vi "bmd101Parser_v1.3.vi"() -> ()   [LabVIEW 2016]
doc: "This example performs writes and reads on a serial port, as directed by the user. You can press the Write and Read buttons, and change the Read Count, while the example is running.\n\nThe parameters set for the serial port must match the parameters of the connected instrument or device. In this example, the Read Count parameter specifies the number of bytes that the serial port reads. If there were more bytes at the port than the specified number, those bytes would not be read. If there were less bytes at the port than the specified number, you would receive a timeout error.\n\nThis example expands upon the flow control options for XON and XOFF, allowing the user to choose those control characters. Also, the user can enable or disable a termination character. Some devices require a termination character in order to identify the end of command strings. Some devices send a termination character to signify the end of data to be read. This example shows how you can end the Read operation once a termination character is detected in the buffer and/or append a termination character at the end of the Write data."
uses:
  C:/Program Files/National Instruments/LabVIEW 2016/examples/Instrument IO/Serial/support/Serial - Settings.ctl
  <vilib>/Instr/_visa.llb/VISA Configure Serial Port (Instr).vi
panel:
  out "Serial Settings:Number of Bytes at Serial Port":u32
  out "size(s)":i32
  out "return count":u32
  in  "Read Count":u32=960
  out "Poor Sensor Quality: \nSensor off":bool
  out "Poor Sensor Quality: \nSensor on":bool
  out "Heart Rate":u16[](array[numeric])
  out "Heart Rate":u8[](graph)
  out "ECG":i16(graph)
  out "Stop Loop":bool
  out "Loop index":i32
  in  "Stop":bool
  in  "Serial Settings":T1={"baud rate"=57600, "data bits"=8, "parity"=enum."None", "stop bits"=10, "flow control"=0} {"flow control" items=["None"=0, "XON/XOFF"=1, "RTS/CTS"=2, "DTR/DSR"=4]; "stop bits" items=["1.0"=10, "1.5"=15, "2.0"=20]; "data bits" min=5 max=8 step=1; "baud rate" items=["75"=75, "110"=110, "134"=134, "150"=150, "300"=300, "600"=600, "1200"=1200, "1800"=1800, "2400"=2400, "4800"=4800, "7200"=7200, "9600"=9600, "14400"=14400, "19200"=19200, "28800"=28800, "38400"=38400, "56000"=56000, "57600"=57600, "115200"=115200, "128000"=128000, "230400"=230400]}
  in  "VISA resource name":refnum<visa-resource-name>="bmd101"
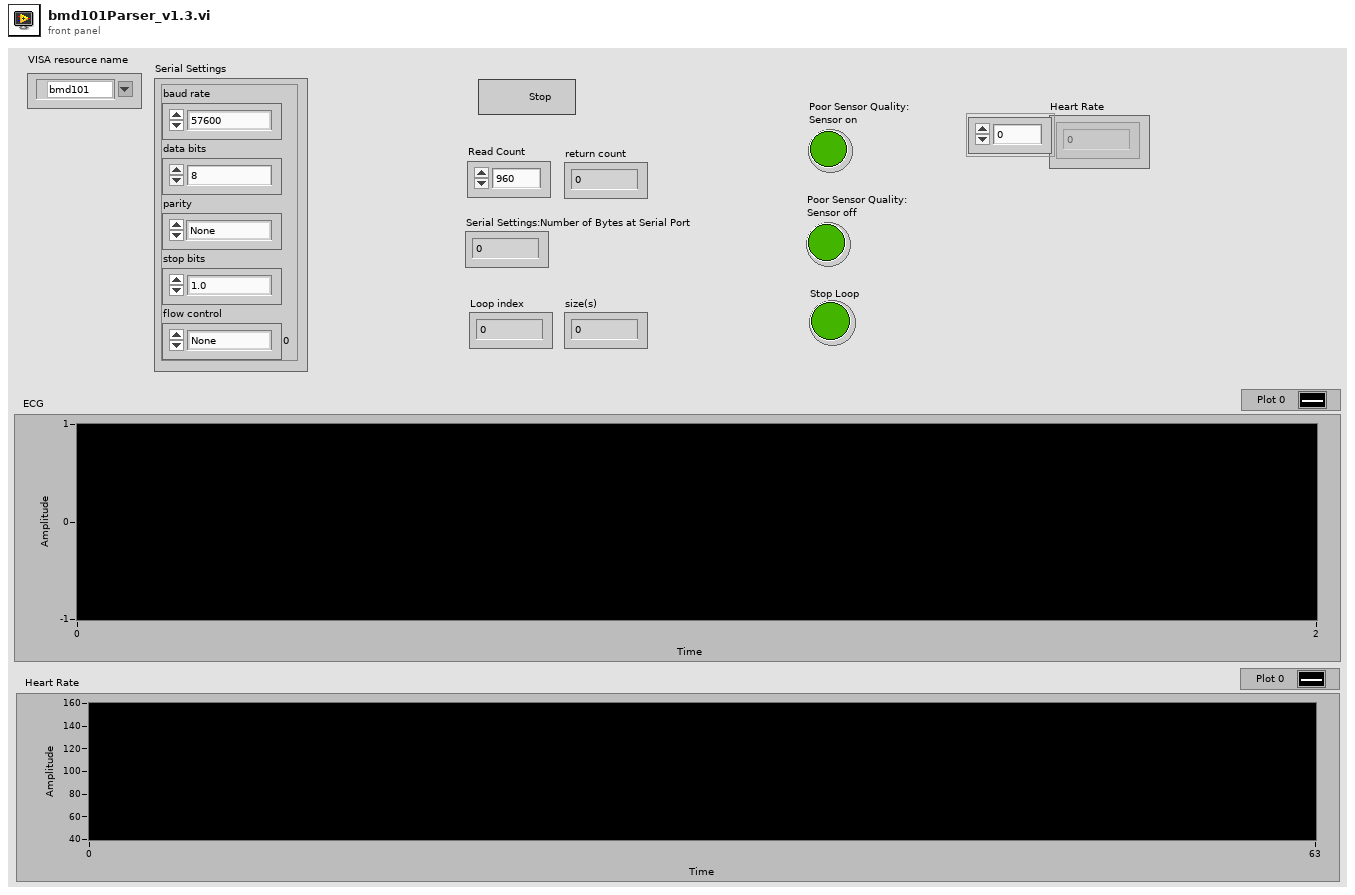
[diagram p1: front panel]
types:
  T1 = typedef "Serial - Settings.ctl" = cluster{"baud rate":u32, "data bits":u16, "parity":enum16{"None", "Odd", "Even", "Mark", "Space"}, "stop bits":u16, "flow control":u16}
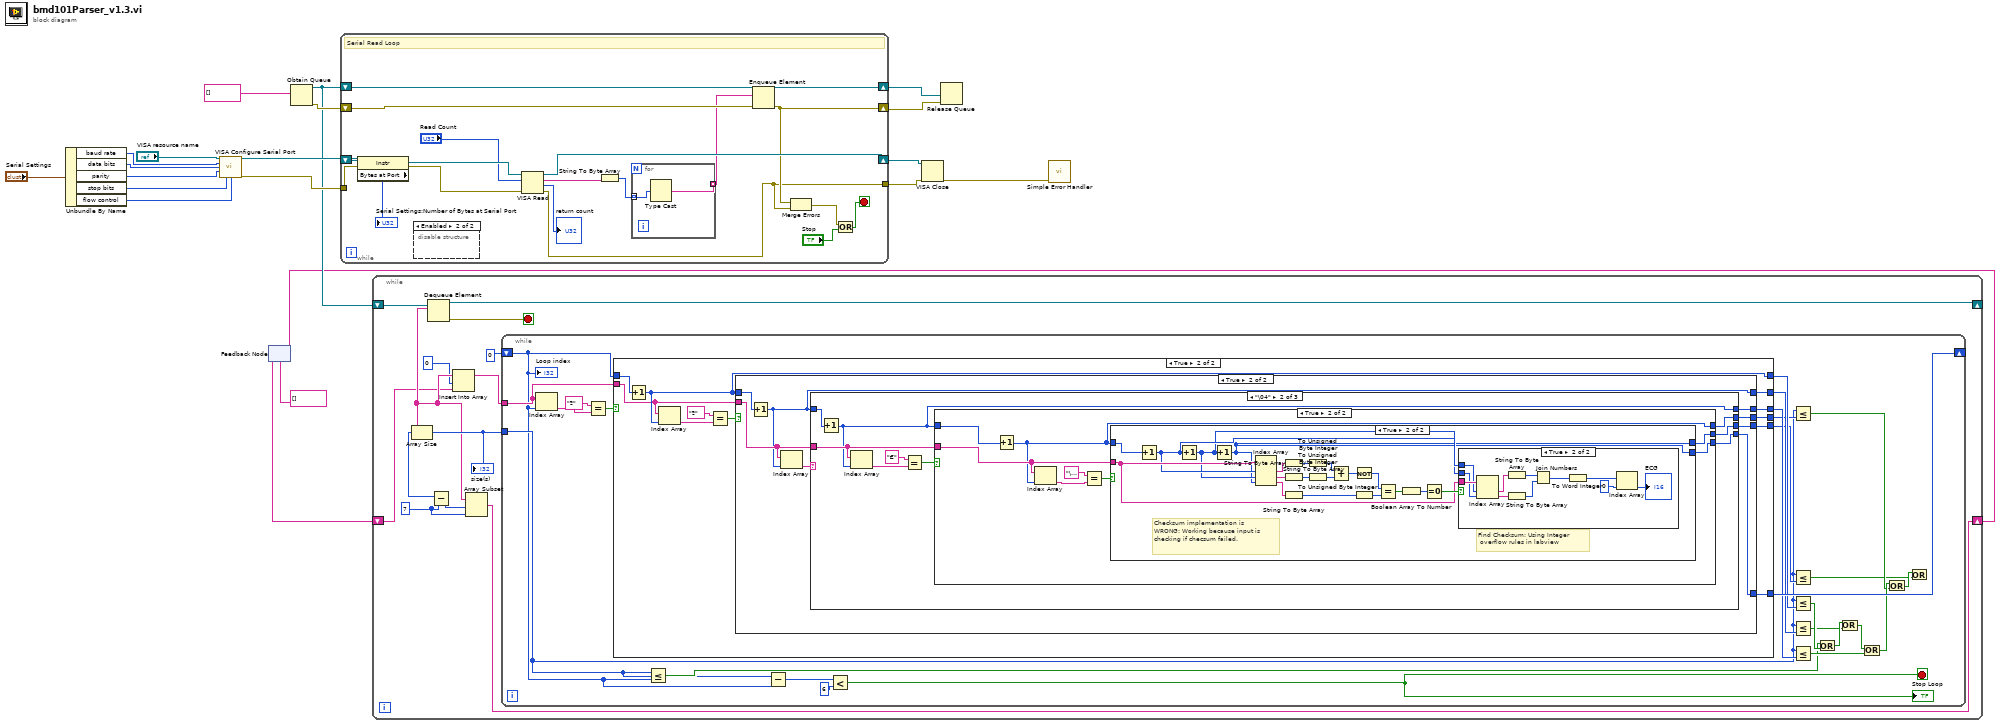
[diagram p0: block diagram]
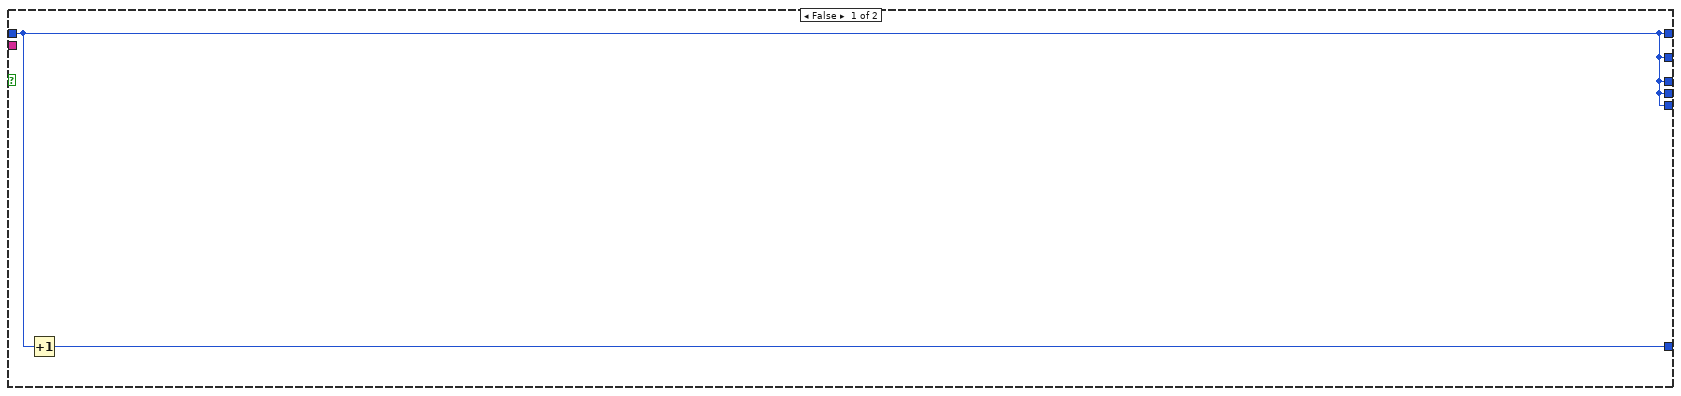
[diagram p2: hidden frame]
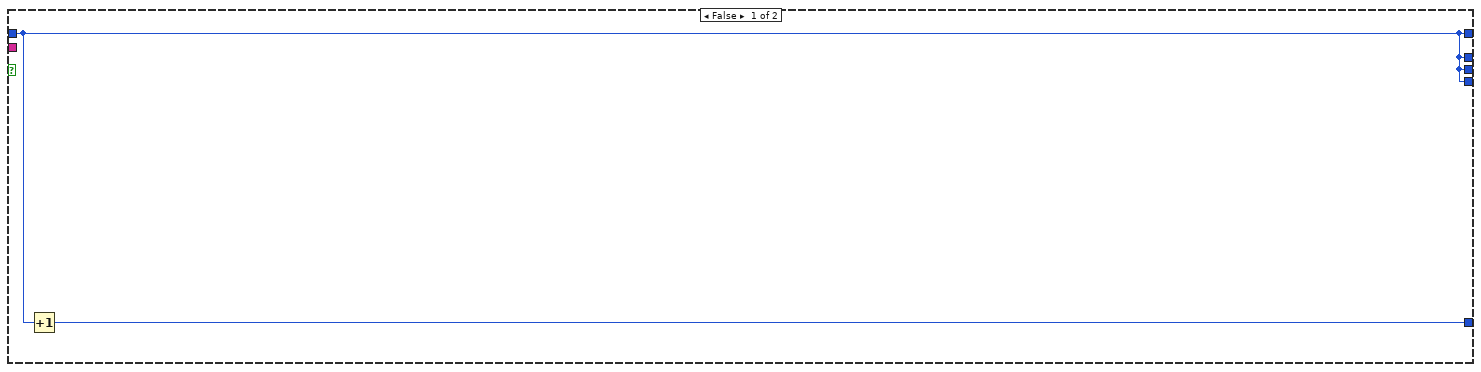
[diagram p3: hidden frame]
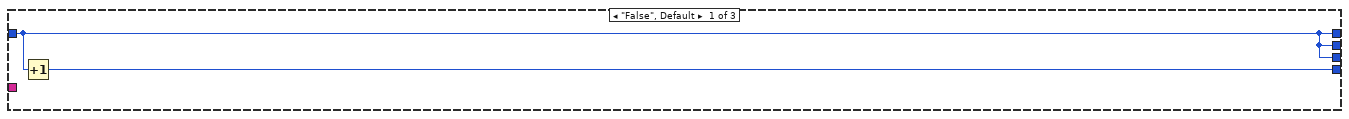
[diagram p4: hidden frame]
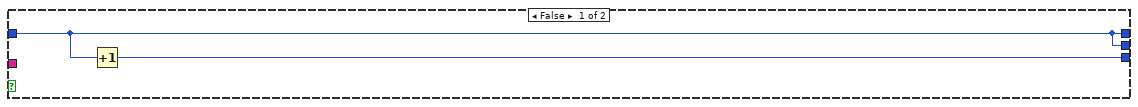
[diagram p5: hidden frame]
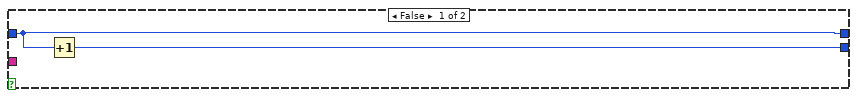
[diagram p6: hidden frame]
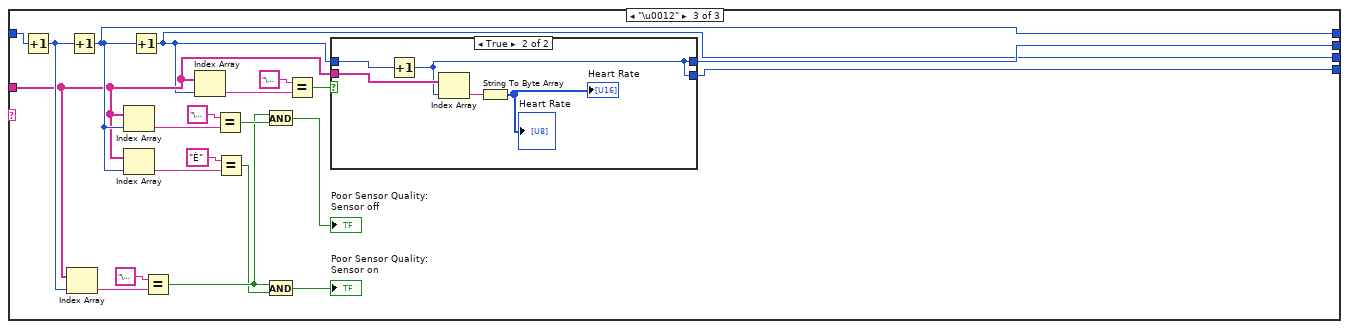
[diagram p8: hidden frame]
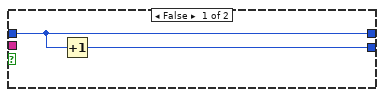
[diagram p9: hidden frame]
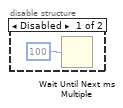
[diagram p10: hidden frame]
diagram:
  n1 = Unbundle By Name("Serial Settings") -> ("baud rate"=w19:u32, "data bits"=w18:u16, "parity"=w17:enum16{"None", "Odd", "Even", "Mark", "Space"}, "stop bits"=w16:u16, "flow control"=w15:u16)
  n2 = call-poly "VISA Configure Serial Port"("VISA resource name"="VISA resource name", "baud rate (9600)"=w19, "data bits (8)"=w18, "parity (0:none)"=w17, "stop bits (10: 1 bit)"=w16, "flow control (0:none)"=w15) -> ("VISA resource name out"=w11:refnum<visa-resource-name>, "error out"=w10:errorcluster)  [unwired: 4 in, 4 out]
  n3 = feedback #1(string[] []) -> (w2:string[])
  n4 = Obtain Queue(element data type=string[] []) -> (queue out=w4:refnum<queue>, error out=w6:errorcluster)  [unwired: 4 in, 1 out]
  n5 = while {
    shift-right: [w36] -> w12
    shift-left: w11 -> [w27]
    tunnel: w10 -> [w25]
    tunnel: [w29] -> w13
    shift-right: [w30] -> w8
    shift-left: w6 -> [w34]
    shift-right: [w31] -> w5
    shift-left: w4 -> [w32]
    stop <- w38 stop-if-true
    # "Serial Read Loop"
    n6 = property class="Instr"(reference=w27, error in=w25) -> (reference out=w26:refnum<visa-resource-name>, error out=w24:errorcluster, "Bytes at Port"=→"Serial Settings:Number of Bytes at Serial Port":u32)
    n7 = disable-structure shown="Enabled" {
      frame Disabled {
        n8 = Wait Until Next ms Multiple(millisecond multiple=u32 100 ("milliseconds to wait")) -> ()  [unwired: 1 out]
      }
      frame Enabled {
      }
    }
    n9 = VISA Read(VISA resource name=w26, byte count="Read Count", error in (no error)=w24) -> (VISA resource name out=w36:refnum<visa-resource-name>, read buffer=w21:string, return count=→"return count":u32, error out=w29:errorcluster)
    n10 = String To Byte Array(string=w21) -> (unsigned byte array=w35:u8[])
    n11 = for {
      tunnel: w35 -> [w42] mode=indexing
      tunnel: [w41] -> w33 mode=indexing
      n12 = Type Cast(x=w42) -> (*(type *) &x=w41:string)  [unwired: 1 in]
    }
    n13 = Enqueue Element(queue=w32, element=w33, error in (no error)=w34) -> (queue out=w31:refnum<queue>, error out=w30:errorcluster)  [unwired: 1 in, 1 out]
    n14 = Merge Errors(w30, w29) -> (w28:errorcluster)
    n15 = Or(x=w28, y="Stop") -> (x .or. y?=w38:bool)
  }
  n16 = while {
    shift-right: [w52] -> _
    shift-left: w4 -> [w53]
    shift-right: [w45] -> w3
    shift-left: w2 -> [w43]
    stop <- w51 stop-if-true
    w48 = 7
    n17 = Dequeue Element(queue=w53) -> (queue out=w52:refnum<queue>, element=w46:string[], error out=w51:errorcluster)  [unwired: 2 in, 1 out]
    n18 = Array Size(array=w46) -> (size(s)=w50:i32)
    "size(s)" <- w50
    n19 = Subtract(x=w50, y=w48) -> (x-y=w49:i32)
    n20 = Insert Into Array(array=w46, index=0, new element=w43) -> (w47:string[])
    n21 = Array Subset(array=w46, index=w49, length=w48) -> (w45:string[])
    n22 = while {
      tunnel: w47 -> [w75]
      shift-right: [w79] -> _
      shift-left: 0 -> [w58]
      tunnel: w50 -> [w59]
      stop <- w55 stop-if-true
      n23 = Index Array(array=w75, index=w58) -> (element=w78:string)
      n24 = Equal?(x="ª", y=w78) -> (x = y?=w76:bool)
      n25 = case shown="True" w76 {
        tunnel: w58 -> [w80 w90]
        tunnel: [w81 w88] -> w79
        tunnel: w75 -> [_ w82]
        tunnel: [w80 w87] -> w74
        tunnel: [w80 w86] -> w72
        tunnel: [w80 w85] -> w69
        tunnel: [w80 w84] -> w66
        tunnel: [w80 w83] -> w63
        frame False {
          n26 = Increment(x=w80) -> (x+1=w81:i32)
        }
        frame True {
          n27 = Increment(x=w90) -> (x+1=w87:i32)
          n28 = Index Array(array=w82, index=w87) -> (element=w92:string)
          n29 = Equal?(x="ª", y=w92) -> (x = y?=w89:bool)
          n30 = case shown="True" w89 {
            tunnel: w87 -> [w93 w96]
            tunnel: [w94 w102] -> w88
            tunnel: w82 -> [_ w101]
            tunnel: [w93 w97] -> w86
            tunnel: [w93 w100] -> w85
            tunnel: [w93 w99] -> w84
            tunnel: [w93 w98] -> w83
            frame False {
              n31 = Increment(x=w93) -> (x+1=w94:i32)
            }
            frame True {
              n32 = Increment(x=w96) -> (x+1=w97:i32)
              n33 = Index Array(array=w101, index=w97) -> (element=w95:string)
              n34 = case shown="\"\\04\"" w95 {
                tunnel: w97 -> [w103 w110 w175]
                tunnel: [w104 w109 w157] -> w102
                tunnel: w101 -> [_ w108 w159]
                tunnel: [w103 w107 w161] -> w100
                tunnel: [w103 w106 w158] -> w99
                tunnel: [w103 w105 w156] -> w98
                frame "False", Default {
                  n35 = Increment(x=w103) -> (x+1=w104:i32)
                }
                frame "\u0004" {
                  n36 = Increment(x=w110) -> (x+1=w107:i32)
                  n37 = Index Array(array=w108, index=w107) -> (element=w111:string)
                  n38 = Equal?(x="€", y=w111) -> (x = y?=w112:bool)
                  n39 = case shown="True" w112 {
                    tunnel: w107 -> [w114 w120]
                    tunnel: [w115 w119] -> w109
                    tunnel: w108 -> [_ w118]
                    tunnel: [w114 w117] -> w106
                    tunnel: [w114 w116] -> w105
                    frame False {
                      n40 = Increment(x=w114) -> (x+1=w115:i32)
                    }
                    frame True {
                      n41 = Increment(x=w120) -> (x+1=w117:i32)
                      n42 = Index Array(array=w118, index=w117) -> (element=w121:string)
                      n43 = Equal?(x="\u0002", y=w121) -> (x = y?=w122:bool)
                      n44 = case shown="True" w122 {
                        tunnel: w117 -> [w124 w129]
                        tunnel: [w125 w126] -> w119
                        tunnel: w118 -> [_ w130]
                        tunnel: [w124 w126] -> w116
                        frame False {
                          n45 = Increment(x=w124) -> (x+1=w125:i32)
                        }
                        frame True {
                          # "Checksum implementation is WRONG: Working because input is checking if checsum failed."
                          # "Find Checksum: Using Integer\n overflow rules in labview"
                          n46 = Increment(x=w129) -> (x+1=w128:i32)
                          n47 = Increment(x=w128) -> (x+1=w127:i32)
                          n48 = Increment(x=w127) -> (x+1=w126:i32)
                          n49 = Index Array(array=w130, index #1=w128, index #2=w127, index #3=w126) -> (element #1=w144:string, element #2=w143:string, element #3=w137:string)
                          n50 = String To Byte Array(string=w144) -> (unsigned byte array=w142:u8[])
                          n51 = String To Byte Array(string=w143) -> (unsigned byte array=w141:u8[])
                          n52 = String To Byte Array(string=w137) -> (unsigned byte array=w136:u8[])
                          n53 = To Unsigned Byte Integer(number=w142) -> (unsigned 8bit integer=w140:u8[])
                          n54 = To Unsigned Byte Integer(number=w141) -> (unsigned 8bit integer=w139:u8[])
                          n55 = Add(x=w140, y=w139) -> (x+y=w138:u8[])
                          n56 = Not(x=w138) -> (.not. x?=w135:u8[])
                          n57 = To Unsigned Byte Integer(number=w136) -> (unsigned 8bit integer=w134:u8[])
                          n58 = Equal?(x=w135, y=w134) -> (x = y?=w133:bool[])
                          n59 = Boolean Array To Number(Boolean array=w133) -> (number=w132:u32)
                          n60 = Equal To 0?(x=w132) -> (x = 0?=w131:bool)
                          n61 = case shown="True" w131 {
                            tunnel: w130 -> [_ w155]
                            tunnel: w128 -> [_ w149]
                            tunnel: w127 -> [_ w148]
                            frame False {
                            }
                            frame True {
                              n62 = Index Array(array=w155, index #1=w149, index #2=w148) -> (element #1=w154:string, element #2=w153:string)
                              n63 = String To Byte Array(string=w154) -> (unsigned byte array=w152:u8[])
                              n64 = String To Byte Array(string=w153) -> (unsigned byte array=w151:u8[])
                              n65 = Join Numbers(hi=w152, lo=w151) -> ((hi.lo)=w150:u16[])
                              n66 = To Word Integer(number=w150) -> (16bit integer=w147:i16[])
                              n67 = Index Array(array=w147, index=0) -> (element=→"ECG":i16)
                            }
                          }
                        }
                      }
                    }
                  }
                }
                frame "\u0012" {
                  n68 = Increment(x=w175) -> (x+1=w171:i32)
                  n69 = Index Array(array=w159, index=w171) -> (element=w174:string)
                  n70 = Increment(x=w171) -> (x+1=w161:i32)
                  n71 = Index Array(array=w159, index=w161) -> (element=w172:string)
                  n72 = Index Array(array=w159, index=w161) -> (element=w169:string)
                  n73 = Increment(x=w161) -> (x+1=w156:i32)
                  n74 = Equal?(x="\u0002", y=w174) -> (x = y?=w166:bool)
                  n75 = Index Array(array=w159, index=w156) -> (element=w162:string)
                  n76 = Equal?(x="\u0000", y=w172) -> (x = y?=w168:bool)
                  n77 = Equal?(x="È", y=w169) -> (x = y?=w165:bool)
                  n78 = And(x=w166, y=w168) -> (x .and. y?=→"Poor Sensor Quality: \nSensor off":bool)
                  n79 = And(x=w166, y=w165) -> (x .and. y?=→"Poor Sensor Quality: \nSensor on":bool)
                  n80 = Equal?(x="\u0003", y=w162) -> (x = y?=w160:bool)
                  n81 = case shown="True" w160 {
                    tunnel: w156 -> [w177 w183]
                    tunnel: w159 -> [_ w182]
                    tunnel: [w177 w181] -> w158
                    tunnel: [w178 w181] -> w157
                    frame False {
                      n82 = Increment(x=w177) -> (x+1=w178:i32)
                    }
                    frame True {
                      n83 = Increment(x=w183) -> (x+1=w181:i32)
                      n84 = Index Array(array=w182, index=w181) -> (element=w180:string)
                      n85 = String To Byte Array(string=w180) -> (unsigned byte array=→"Heart Rate" →"Heart Rate":u8[])
                    }
                  }
                }
              }
            }
          }
        }
      }
      n86 = Less Or Equal?(x=w59, y=w58) -> (x <= y?=w60:bool)
      n87 = Subtract(x=w59, y=w58) -> (x-y=w57:i32)
      n88 = Less?(x=w57, y=6) -> (x < y?=w55:bool)
      "Stop Loop" <- w55
      n89 = Less Or Equal?(x=w59, y=w66) -> (x <= y?=w64:bool)
      n90 = Less Or Equal?(x=w59, y=w63) -> (x <= y?=w61:bool)
      n91 = Less Or Equal?(x=w59, y=w74) -> (x <= y?=w73:bool)
      n92 = Less Or Equal?(x=w59, y=w72) -> (x <= y?=w70:bool)
      n93 = Less Or Equal?(x=w59, y=w69) -> (x <= y?=w67:bool)
      n94 = Or(x=w60, y=w73) -> (x .or. y?=w71:bool)
      n95 = Or(x=w71, y=w70) -> (x .or. y?=w68:bool)
      n96 = Or(x=w68, y=w67) -> (x .or. y?=w65:bool)
      n97 = Or(x=w65, y=w64) -> (x .or. y?=w62:bool)
      n98 = Or(x=w62, y=w61) -> ()  [unwired: 1 out]
      "Loop index" <- w58
    }
  }
  n99 = feedback-in #1(w3) -> ()
  n100 = VISA Close(VISA resource name=w12, error in (no error)=w13) -> (error out=w9:errorcluster)
  n101 = Release Queue(queue=w5, error in (no error)=w8) -> ()  [unwired: 1 in, 3 out]
  n102 = call <vilib>:"Simple Error Handler.vi"("error in (no error)"=w9) -> ()  [unwired: 1 in, 8 out]
